vi "ViHandler.SetStartTime.vi"(8 "error in (no error)":errorcluster, 10 "Start Time":timestamp, 11 "ViHandler in":refnum<class "ViHandler.lvclass">) -> (0 "error out":errorcluster, 3 "ViHandler out":refnum<class "ViHandler.lvclass">)   [LabVIEW 2016, in "ViHandler.lvclass"]
uses:
  ViHandler.lvclass
  ViHandler.lvclass/ViHandler.ctl
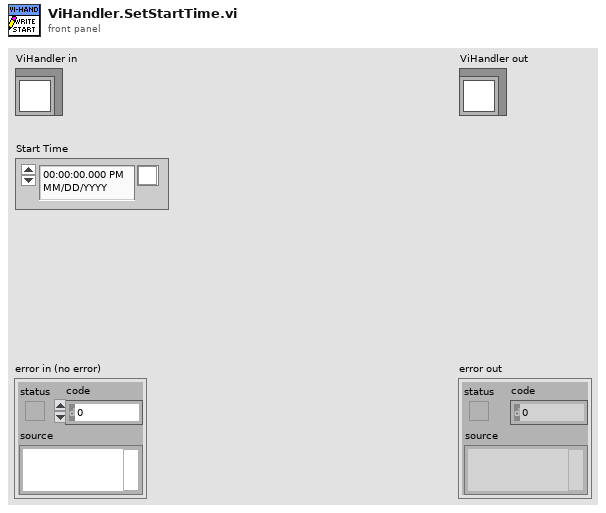
[diagram p1: front panel]
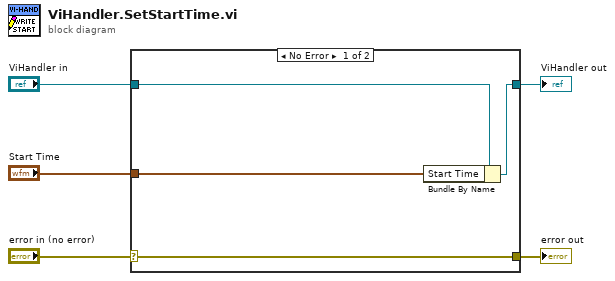
[diagram p0: block diagram]
diagram:
  n1 = case shown="No Error" "error in (no error)" {
    selector: "error in (no error)" -> [w9 w10]
    tunnel: [w9 w10] -> w4
    tunnel: [w7 w11] -> w2
    tunnel: "ViHandler in" -> [w8 w11]
    tunnel: "Start Time" -> [w6 _]
    frame No Error {
      n2 = Bundle By Name(cluster=w8, "Start Time"=w6) -> (w7:refnum<class "ViHandler.lvclass">)
    }
    frame Error {
    }
  }
  "error out" <- w4
  "ViHandler out" <- w2
